vi "Flush Queue.vi"(8 "error in (no error)":errorcluster) -> (0 "error out":errorcluster, 3 "remaining elements":T1[](array[typedef]))   [LabVIEW 2020, in "UI.lvlib"]
uses:
  UI.lvlib
  Module Support/Queue FGV Action.ctl
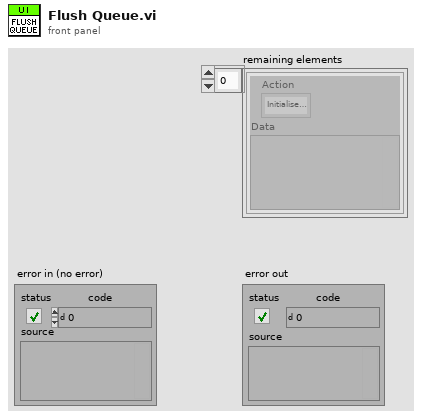
[diagram p1: front panel]
types:
  T1 = typedef "Module Data Cluster.ctl" = cluster{"Action":T2, "Data":variant}
  T2 = typedef "Module Action.ctl" = enum16{"Initialise Module", "Connect", "Setup", "Pause", "Start", "Stop", "Wait: Time Elapsed", "Error", "Exit"}
  T3 = typedef "UI.lvlib/Queue FGV Action.ctl" = enum16{"Get", "Set", "Release"}
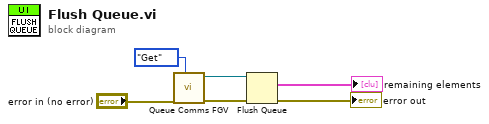
[diagram p0: block diagram]
diagram:
  n1 = call "Queue Comms FGV.vi"("Action"=Queue_FGV_Action."Get", "error in (no error)"="error in (no error)") -> ("error out"=w5:errorcluster, "queue In"=w3:refnum<queue>)  [unwired: 8 in]
  n2 = Flush Queue(queue=w3, error in (no error)=w5) -> (remaining elements=→"remaining elements":T1[], error out=→"error out":errorcluster)  [unwired: 1 out]
